vi "Add Time Date String.vi"(9 "Prefix":string) -> (3 "String out":string)   [LabVIEW 2012]
doc: "Adds a time-date string to incomming string"
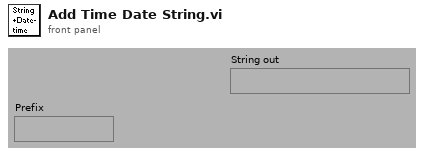
[diagram p1: front panel]
types:
  T1 = cluster{"second":i32, "minute":i32, "hour":i32, "day of month":i32, "month":i32, "year":i32, "day of week":i32, "day of year":i32, "is DST":i32}
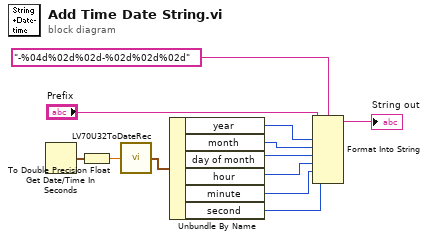
[diagram p0: block diagram]
diagram:
  n1 = Get Date/Time In Seconds() -> (seconds since 1Jan1904=w12:timestamp)
  n2 = To Double Precision Float(number=w12) -> (double precision float=w5:dbl)
  n3 = call <vilib>:"LV70U32ToDateRec.vi"("Time"=w5) -> ("date time rec"=w11:T1)
  n4 = Unbundle By Name(w11) -> ("year"=w10:i32, "month"=w9:i32, "day of month"=w8:i32, "hour"=w7:i32, "minute"=w4:i32, "second"=w1:i32)
  n5 = Format Into String(format string="-%04d%02d%02d-%02d%02d%02d" ("Format String"), initial string="Prefix", w10, w9, w8, w7, w4, w1) -> (resulting string=→"String out":string)  [unwired: 1 in, 1 out]
